vi "IsmaCTRL_single.vi"(1 "FR_manual":dbl, 2 "tube selector":dbl, 8 "Manual":bool, 12 "Reset":bool, 14 "Pause":bool, 16 "Setpoint_W   /   Setpoint_T":dbl[][](array[numeric]), 18 "Enable":bool, 19 "Scale":dbl[](array[numeric])) -> (0 "timeChange":dbl, 3 "Boolean 9":bool, 4 "Boolean":bool, 5 "Boolean 2":bool, 6 "Total target":dbl, 7 "Boolean 3":bool, 9 "Boolean 4":bool, 10 "lastAmount":dbl, 11 "step":dbl, 13 "Boolean 5":bool, 15 "Boolean 6":bool, 17 "Boolean 7":bool, 20 "FR":dbl, 21 "RPM":dbl, 22 "Weight":dbl, 23 "elapsed":dbl, 24 "time_to_target":dbl, 25 "pumpCTRL":dbl, 26 "Target_step":dbl, 27 "Boolean 8":bool)   [LabVIEW 2017]
uses:
  BERTTA/x64/Debug/BERTTA.dll
panel:
  out "paramsIn":dbl[](array[numeric])
  out "paramsOut":dbl[](array[numeric])
  # "STOP"
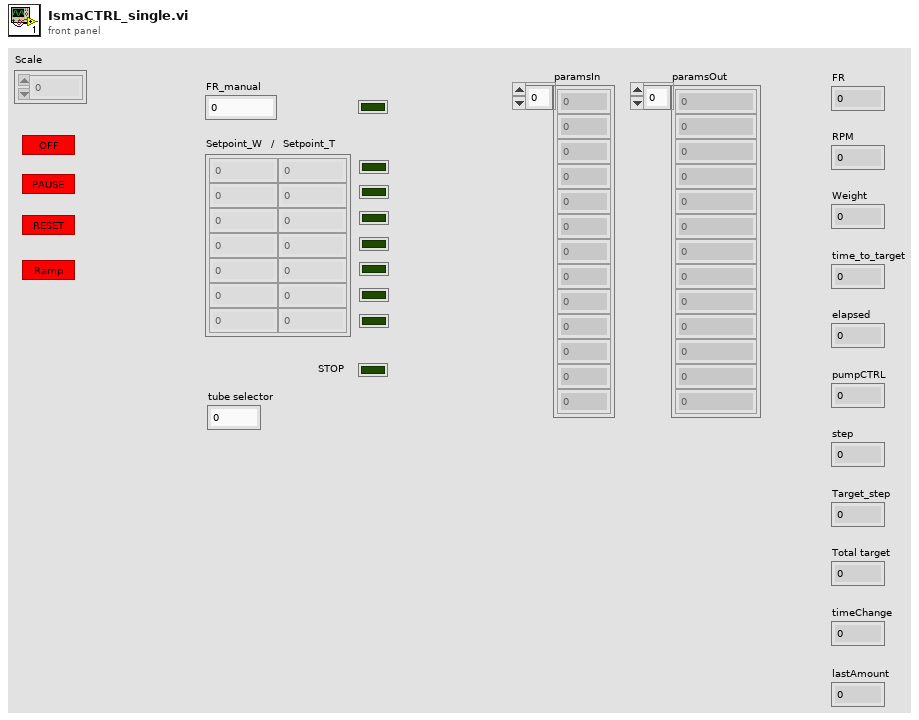
[diagram p1: front panel]
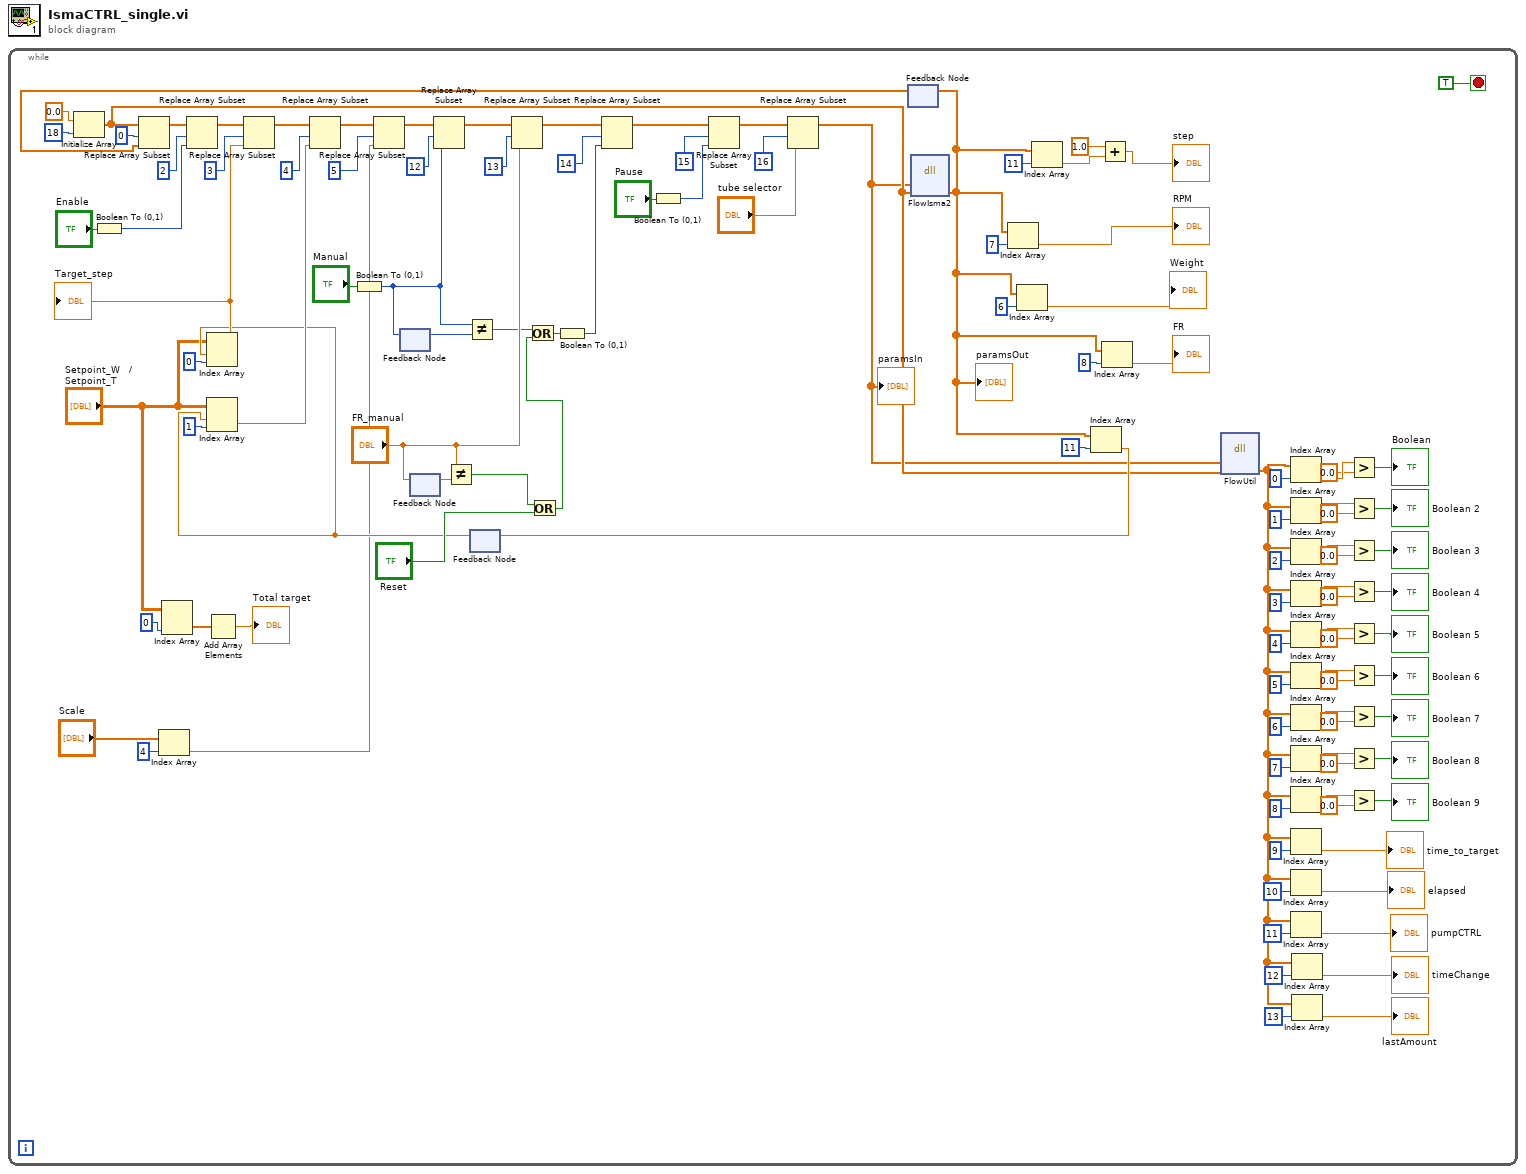
[diagram p0: block diagram]
diagram:
  n1 = while {
    stop <- TRUE stop-if-true
    n2 = Initialize Array(0.0 ("element"), 18 ("dimension size")) -> (w23:dbl[])
    n3 = Boolean To (0,1)(Boolean="Enable") -> (0, 1=w91:i16)
    n4 = Index Array(array="Scale", index=4) -> (element=w20:dbl)
    n5 = Index Array(array="Setpoint_W   /   Setpoint_T", index (col)=0 ("index (row)")) -> (element=w10:dbl[])  [unwired: 1 in]
    n6 = Add Array Elements(numeric array=w10) -> (sum=→"Total target":dbl)
    n7 = Boolean To (0,1)(Boolean="Manual") -> (0, 1=w82:i16)
    n8 = feedback #1() -> (w83:i16)  [unwired: 1 in]
    n9 = feedback-in #1(w82) -> ()
    n10 = feedback #2() -> (w86:dbl)  [unwired: 1 in]
    n11 = feedback-in #2("FR_manual") -> ()
    n12 = Not Equal?(x="FR_manual", y=w86) -> (x != y?=w85:bool)
    n13 = Not Equal?(x=w82, y=w83) -> (x != y?=w79:bool)
    n14 = feedback #3() -> (w66:dbl)  [unwired: 1 in]
    n15 = Index Array(array="Setpoint_W   /   Setpoint_T", index (row)=w66, index (col)=0 ("disabled index (col)")) -> (element=w71:dbl)
    "Target_step" <- w71
    n16 = Index Array(array="Setpoint_W   /   Setpoint_T", index (row)=w66, index (col)=1 ("disabled index (col)")) -> (element=w69:dbl)
    n17 = Or(x=w85, y="Reset") -> (x .or. y?=w78:bool)
    n18 = Or(x=w79, y=w78) -> (x .or. y?=w81:bool)
    n19 = Boolean To (0,1)(Boolean=w81) -> (0, 1=w80:i16)
    n20 = Boolean To (0,1)(Boolean="Pause") -> (0, 1=w73:i16)
    n21 = feedback #4() -> (w99:dbl[])  [unwired: 1 in]
    n22 = Replace Array Subset(array=w23, new element=w99, index=0) -> (w98:dbl[])
    n23 = Replace Array Subset(array=w98, new element=w91, index=2) -> (w108:dbl[])
    n24 = Replace Array Subset(array=w108, new element=w71, index=3) -> (w106:dbl[])
    n25 = Replace Array Subset(array=w106, new element=w69, index=4) -> (w104:dbl[])
    n26 = Replace Array Subset(array=w104, new element=w20, index=5) -> (w96:dbl[])
    n27 = Replace Array Subset(array=w96, new element=w82, index=12) -> (w93:dbl[])
    n28 = Replace Array Subset(array=w93, new element="FR_manual", index=13) -> (w88:dbl[])
    n29 = Replace Array Subset(array=w88, new element=w80, index=14) -> (w75:dbl[])
    n30 = Replace Array Subset(array=w75, new element=w73, index=15) -> (w7:dbl[])
    n31 = Replace Array Subset(array=w7, new element="tube selector", index=16) -> (w6:dbl[])
    "paramsIn" <- w6
    n32 = dll-call lib="C:/Users/shresplab/OneDrive - Kemira Oyj/Documents/GitHub/Bertta/BERTTA/x64/Debug/BERTTA.dll" fn="FlowIsma2"("paramsIn"=w6, "paramsOut"=w23) -> ("paramsOut"=w17:dbl[])  [unwired: 5 in, 2 out]
    "paramsOut" <- w17
    n33 = feedback-in #4(w17) -> ()
    n34 = Index Array(array=w17, index=7) -> (element=→"RPM":dbl)
    n35 = Index Array(array=w17, index=6) -> (element=→"Weight":dbl)
    n36 = Index Array(array=w17, index=11) -> (element=w16:dbl)
    n37 = Index Array(array=w17, index=11) -> (element=w67:dbl)
    n38 = feedback-in #3(w67) -> ()
    n39 = Add(x=1.0, y=w16) -> (x+y=→"step":dbl)
    n40 = Index Array(array=w17, index=8) -> (element=→"FR":dbl)
    n41 = dll-call lib="C:/Users/shresplab/OneDrive - Kemira Oyj/Documents/GitHub/Bertta/BERTTA/x64/Debug/BERTTA.dll" fn="FlowUtil"("paramsIn"=w6, "paramsOut2"=w23) -> ("paramsOut2"=w1:dbl[])  [unwired: 5 in, 2 out]
    n42 = Index Array(array=w1, index=0) -> (element=w53:dbl)
    n43 = Index Array(array=w1, index=1) -> (element=w52:dbl)
    n44 = Index Array(array=w1, index=2) -> (element=w51:dbl)
    n45 = Index Array(array=w1, index=3) -> (element=w50:dbl)
    n46 = Index Array(array=w1, index=4) -> (element=w49:dbl)
    n47 = Index Array(array=w1, index=5) -> (element=w48:dbl)
    n48 = Index Array(array=w1, index=6) -> (element=w47:dbl)
    n49 = Index Array(array=w1, index=7) -> (element=w46:dbl)
    n50 = Index Array(array=w1, index=8) -> (element=w45:dbl)
    n51 = Index Array(array=w1, index=9) -> (element=→"time_to_target":dbl)
    n52 = Index Array(array=w1, index=10) -> (element=→"elapsed":dbl)
    n53 = Index Array(array=w1, index=11) -> (element=→"pumpCTRL":dbl)
    n54 = Index Array(array=w1, index=12) -> (element=→"timeChange":dbl)
    n55 = Index Array(array=w1, index=13) -> (element=→"lastAmount":dbl)
    n56 = Greater?(x=w53, y=0.0) -> (0:→"Boolean":bool)
    n57 = Greater?(x=w52, y=0.0) -> (0:→"Boolean 2":bool)
    n58 = Greater?(x=w51, y=0.0) -> (0:→"Boolean 3":bool)
    n59 = Greater?(x=w50, y=0.0) -> (0:→"Boolean 4":bool)
    n60 = Greater?(x=w49, y=0.0) -> (0:→"Boolean 5":bool)
    n61 = Greater?(x=w48, y=0.0) -> (0:→"Boolean 6":bool)
    n62 = Greater?(x=w47, y=0.0) -> (0:→"Boolean 7":bool)
    n63 = Greater?(x=w46, y=0.0) -> (0:→"Boolean 8":bool)
    n64 = Greater?(x=w45, y=0.0) -> (0:→"Boolean 9":bool)
  }
